vi "古田户外一体站流程质控自动启动.vi"(6 "CODMn量程切换":enum32{"H", "L", "AUTO"}(ring)=enum."AUTO", 8 "总磷量程切换":enum32{"H", "L", "AUTO"}(ring)=enum."AUTO", 9 "总氮量程切换":enum32{"H", "L", "AUTO"}(ring)=enum."AUTO", 10 "氨氮量程切换":enum32{"H", "L", "AUTO"}(ring)=enum."AUTO", 11 "参数":T1={"是否启用仪器"=FALSE, "CODMn"={"启动测量模式"={"测量模式"=enum."水样测量"}, "确定按钮"=TRUE}, "启动模块"={"氨氮"=FALSE, "总磷"=FALSE, "总氮"=FALSE, "COD"=FALSE}, "常规启动"=FALSE, "直接启动"=FALSE}) -> ()   [LabVIEW 2016, in "质控单元.lvlib"]
uses:
  PLC/PLC.lvlib
panel:
  out "枚举 2":enum16{"初始化", "采配水启动", "等待", "配水", "排水", "结束"}(ring)
  out "枚举":enum16{"初始化", "采配水启动", "等待", "配水", "排水", "结束"}(ring)
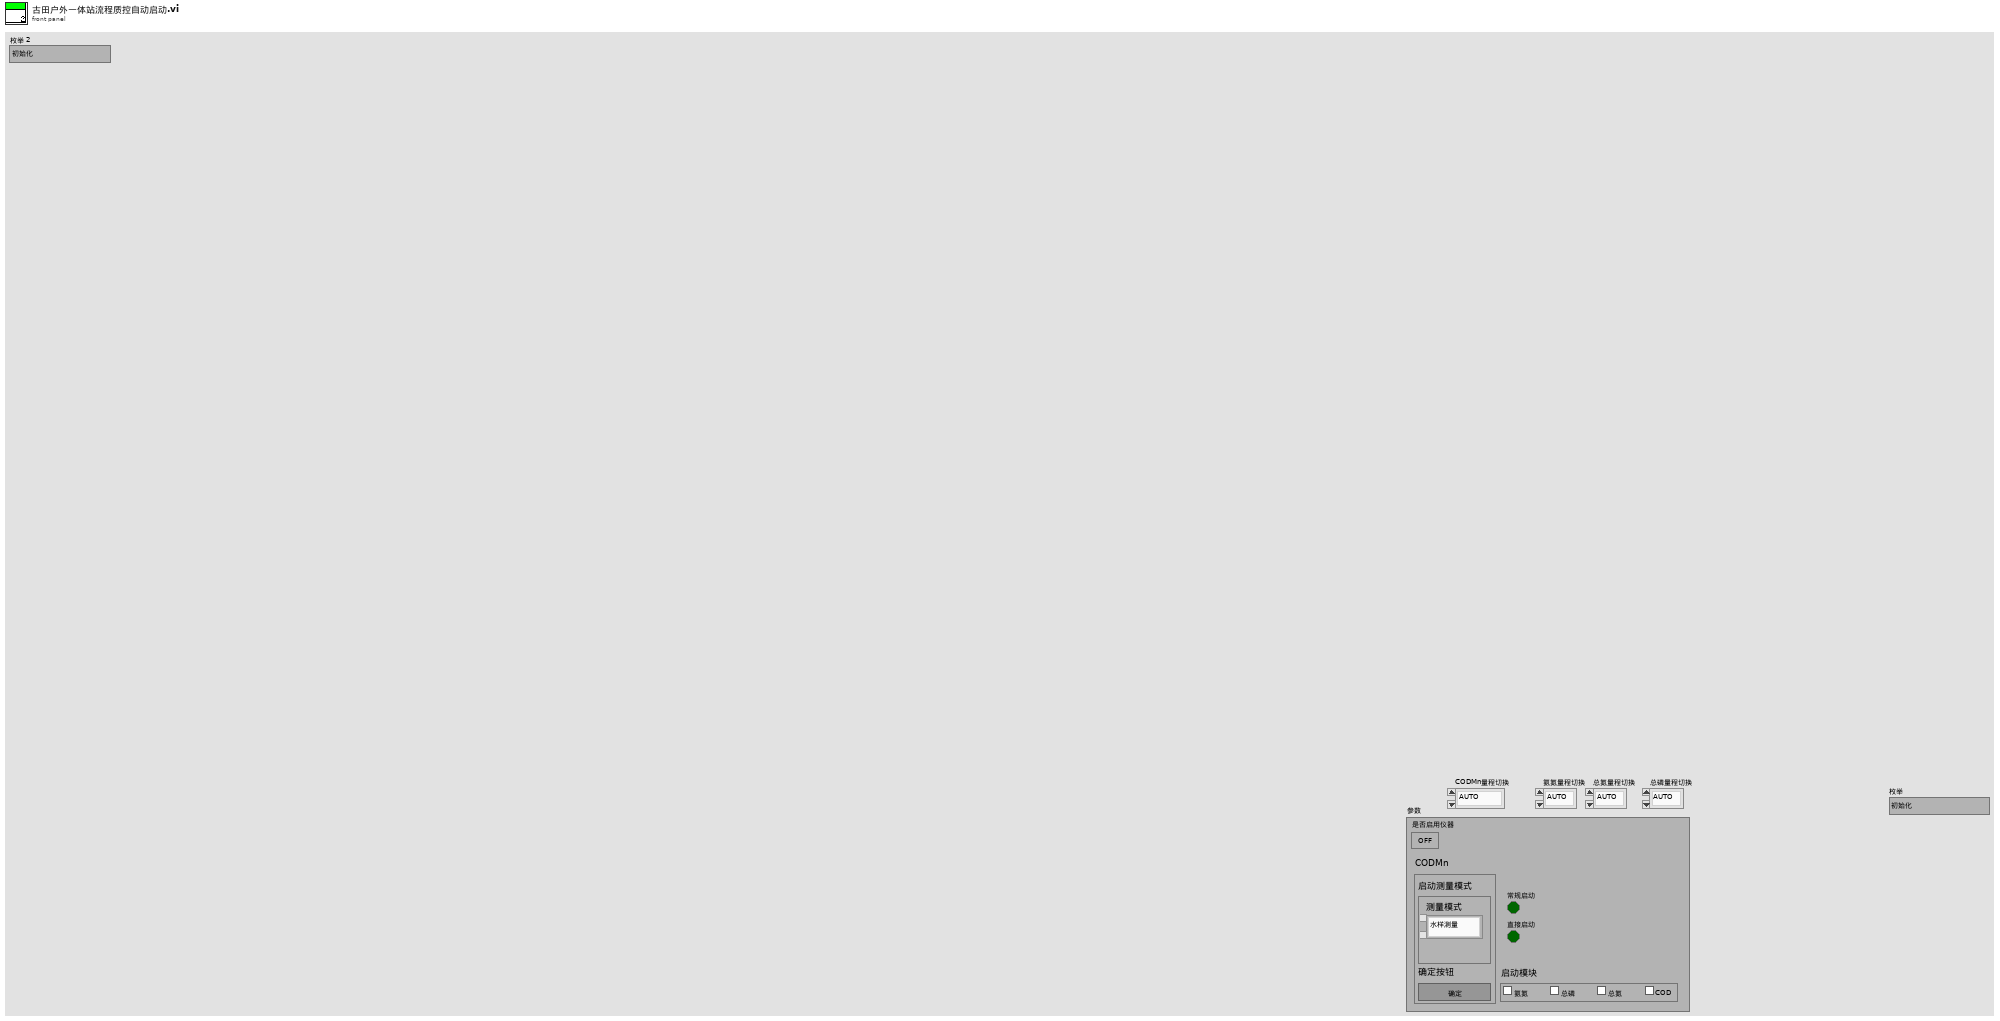
[diagram p1: front panel]
types:
  T1 = cluster{"是否启用仪器":bool, "CODMn":cluster{"启动测量模式":cluster{"测量模式":enum16{"水样测量", "标样核查", "加标回收", "平行样", "校零", "校标"}}, "确定按钮":bool}, "启动模块":cluster{"氨氮":bool, "总磷":bool, "总氮":bool, "COD":bool}, "常规启动":bool, "直接启动":bool}
  T2 = cluster{"命令":string, cluster{"starting address":u16, "holding register value":u16}}
  T3 = cluster{"R0":i16, "R1":i16, "R2":i16, "R3":i16, "R4":i16, "R5":i16, "R6":i16, "R7":i16, "R8":i16, "R9":i16, "R10":i16, "R11":i16, "R12":i16, "R13":i16, "R14":i16, "R15":i16, "R16":i16, "R17":i16, "R18":i16, "R19":i16, "R20":i16, "R21":i16, "R22":i16, "R23":i16, "R24":i16, "R25":i16}
  T4 = enum32{"Bad", "Idle", "Run top level", "Running"}
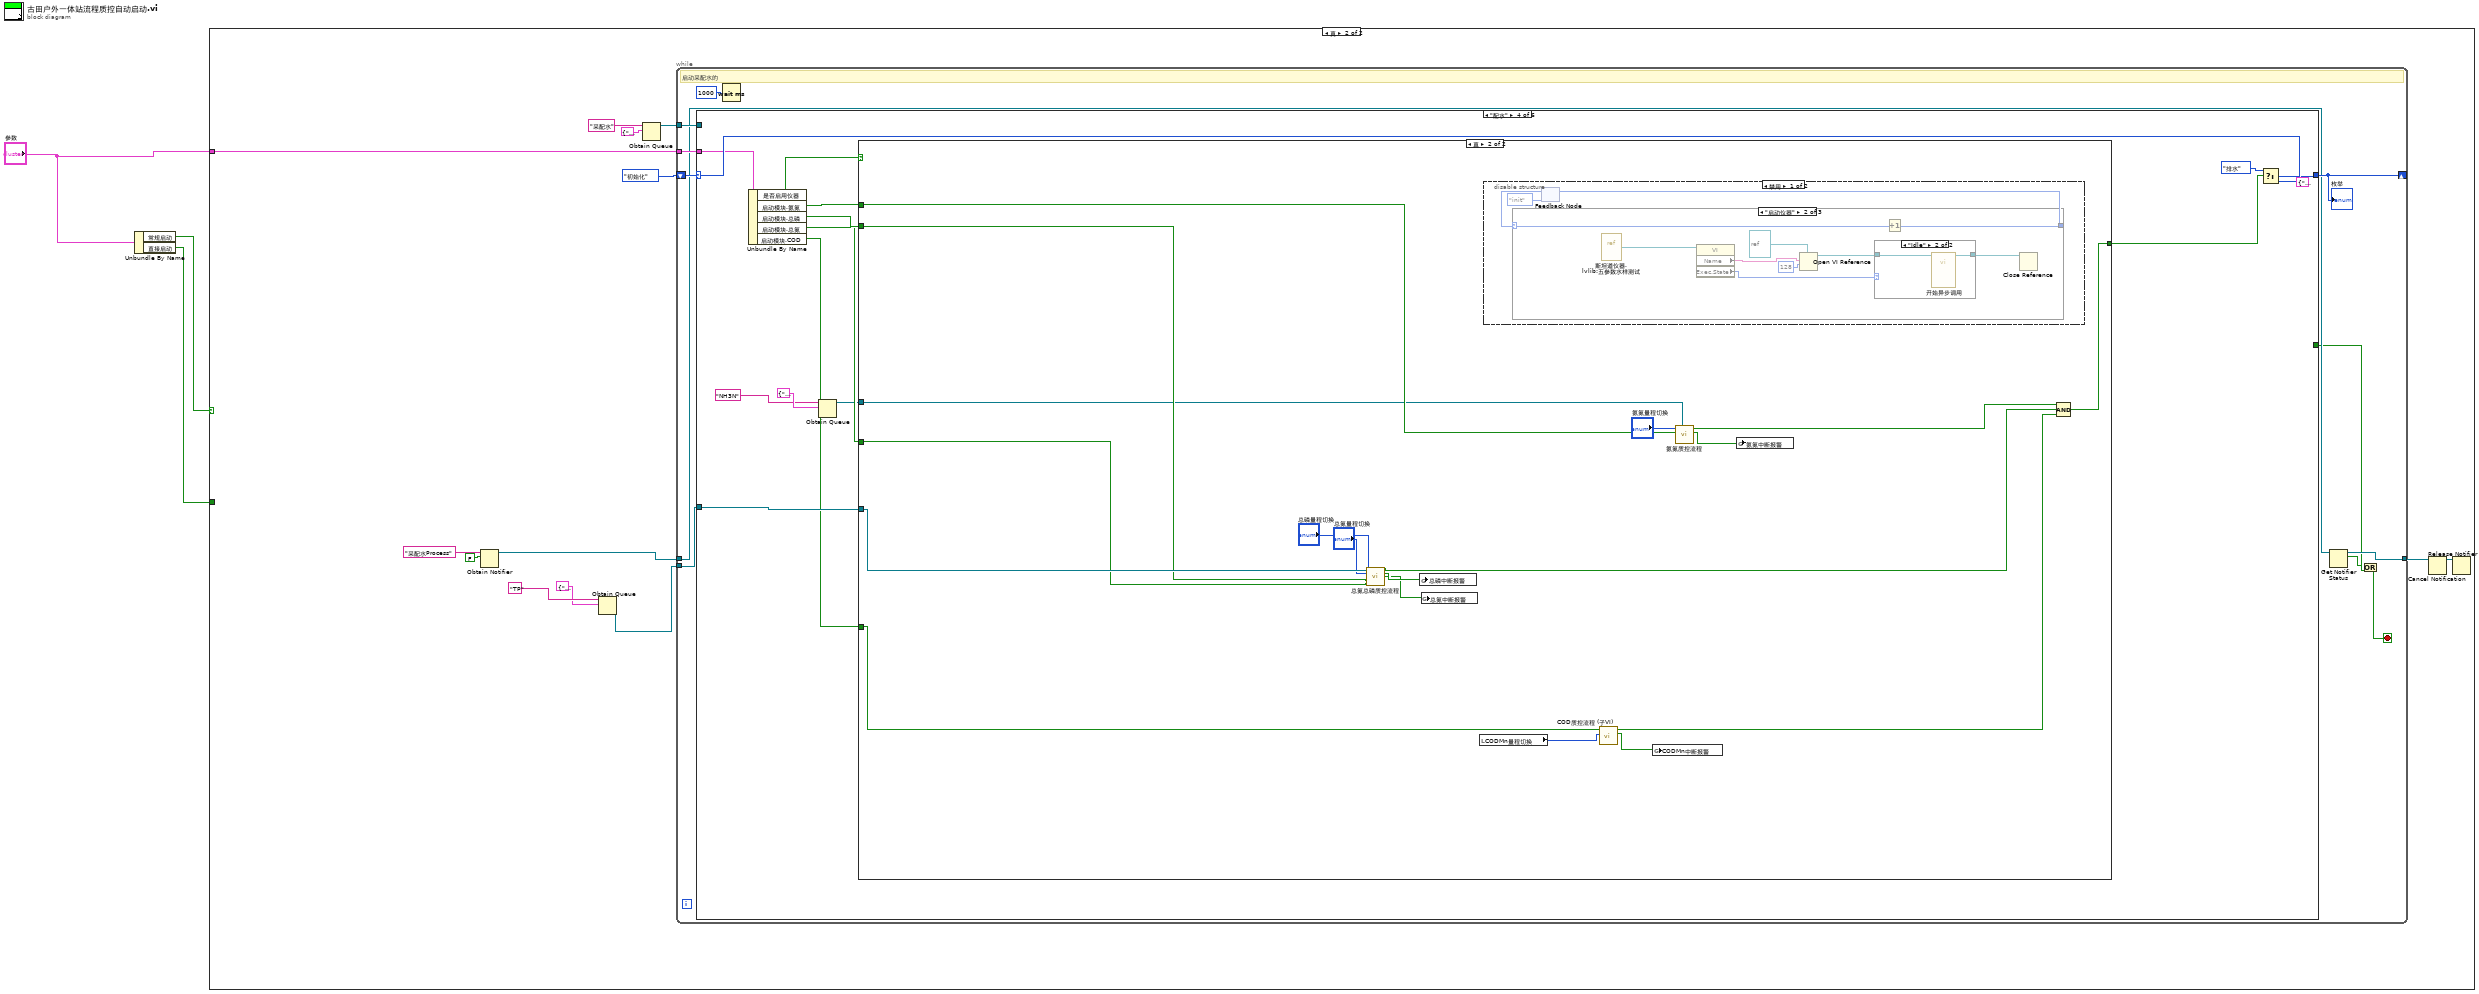
[diagram p0: block diagram]
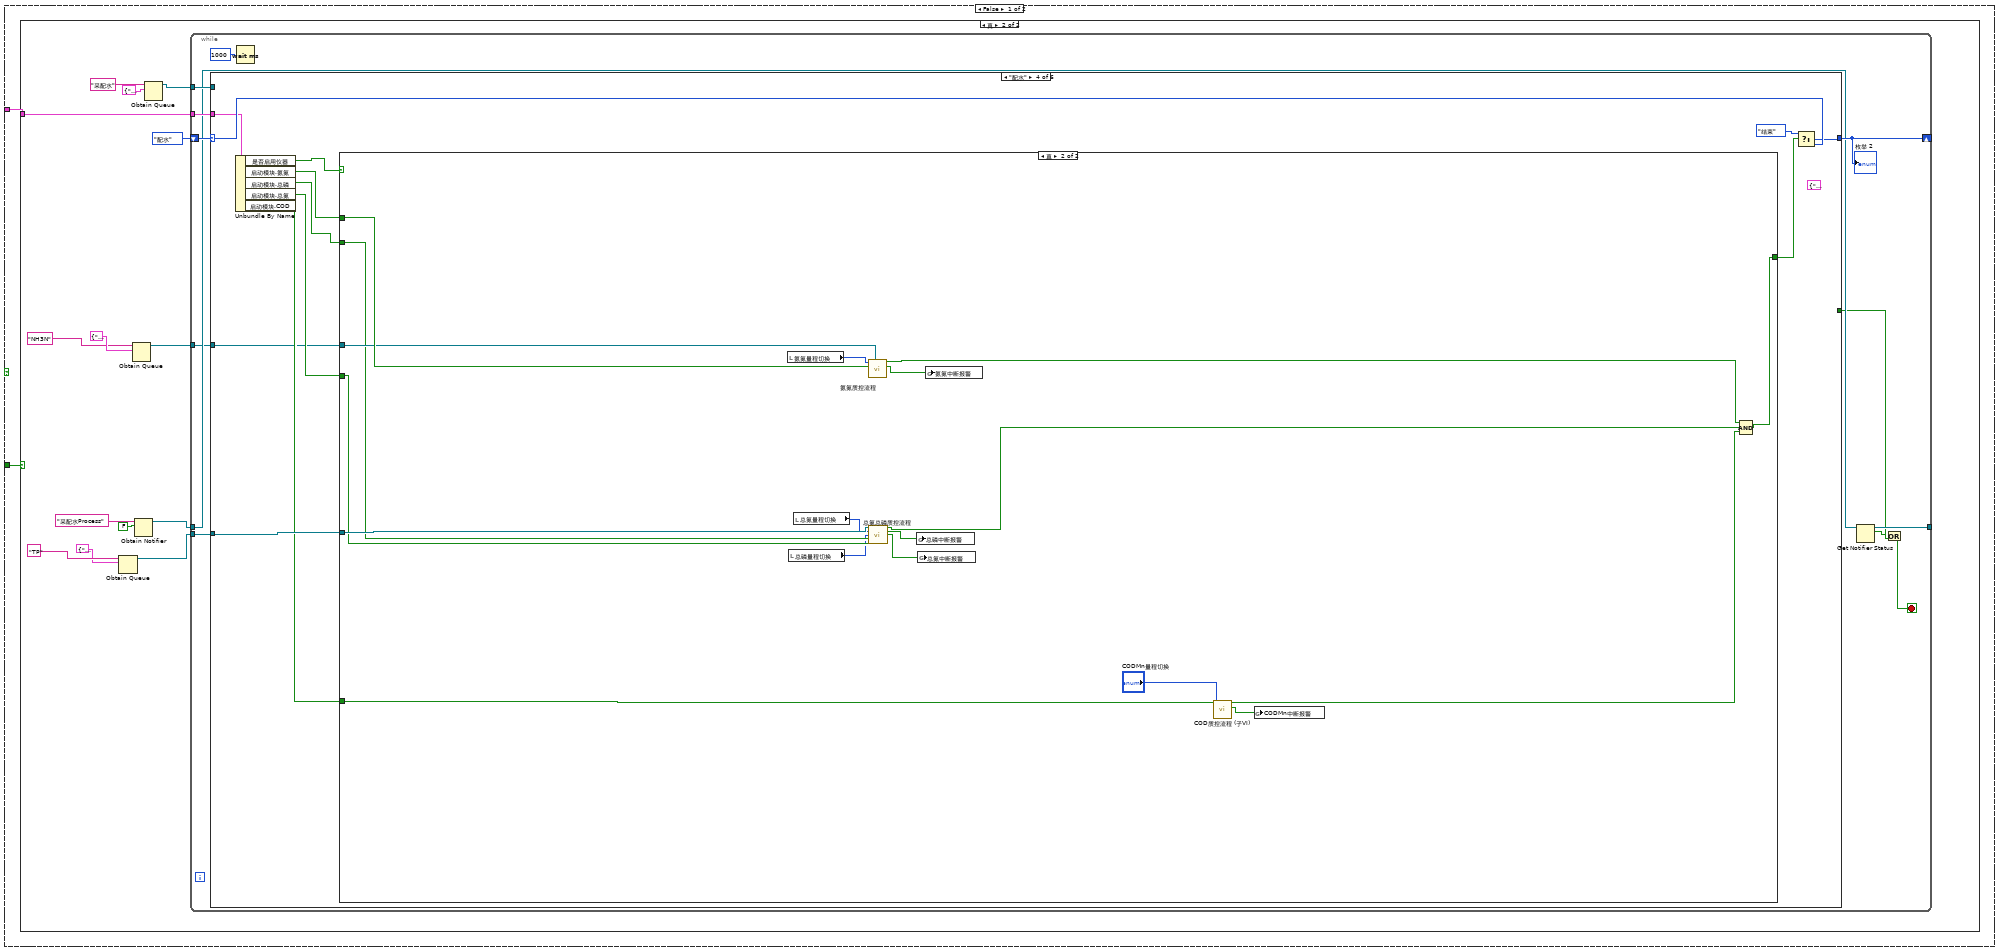
[diagram p2: hidden frame]
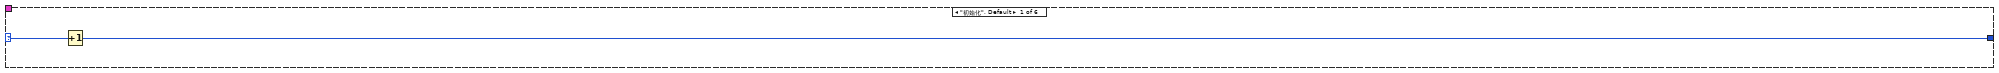
[diagram p4: hidden frame]
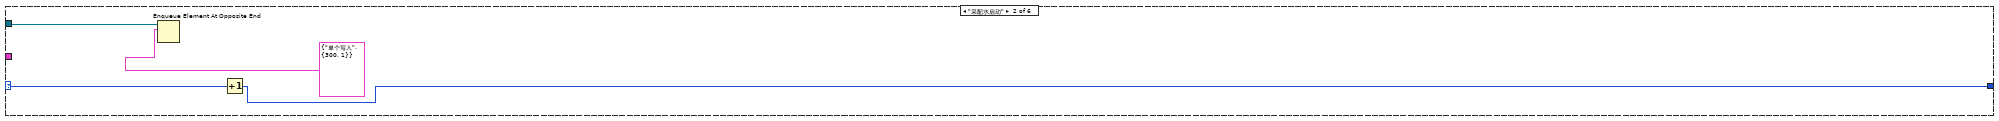
[diagram p5: hidden frame]
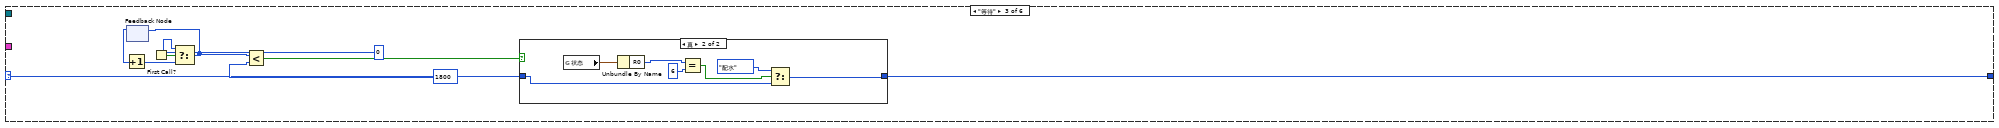
[diagram p6: hidden frame]
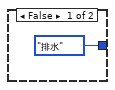
[diagram p7: hidden frame]
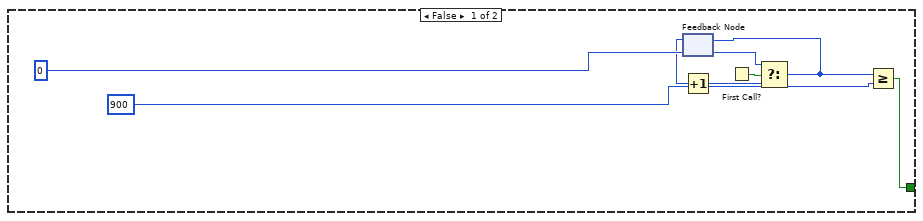
[diagram p8: hidden frame]
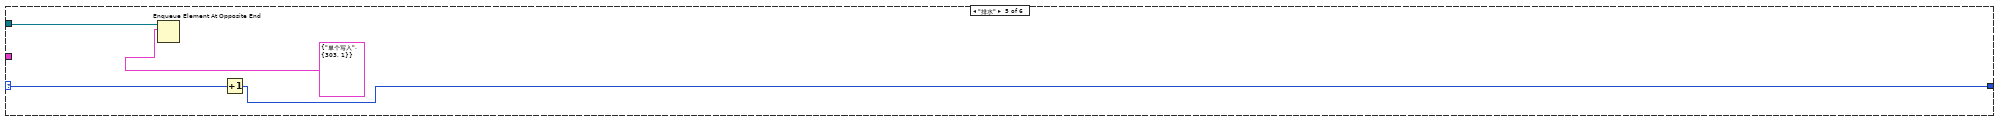
[diagram p9: hidden frame]
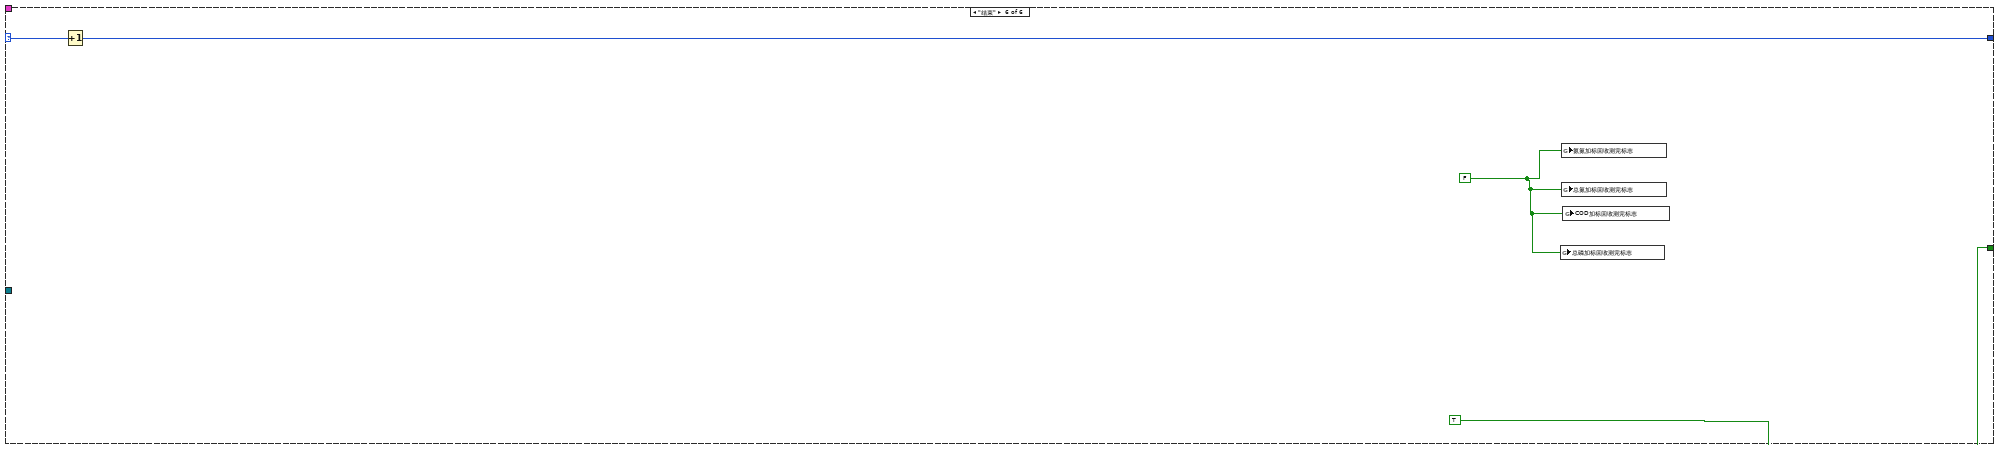
[diagram p10: hidden frame]
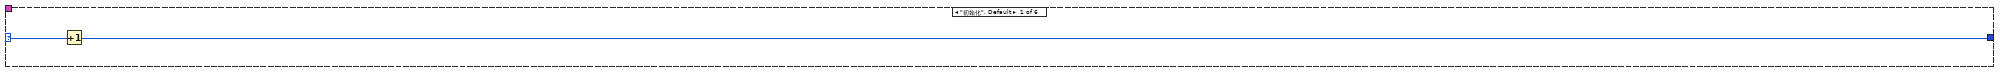
[diagram p11: hidden frame]
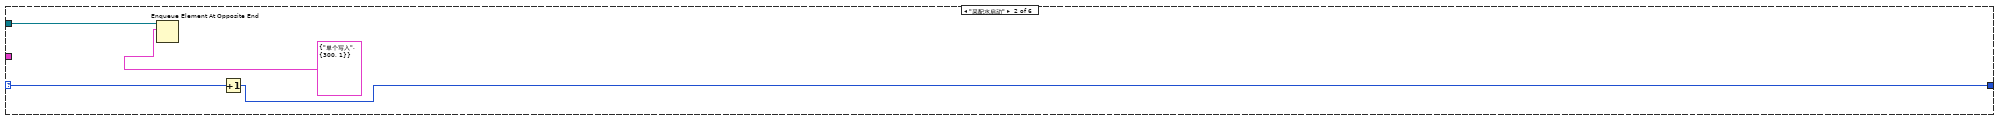
[diagram p12: hidden frame]
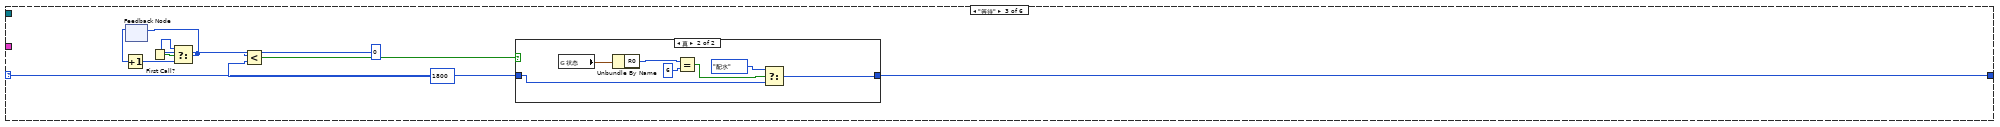
[diagram p13: hidden frame]
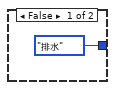
[diagram p14: hidden frame]
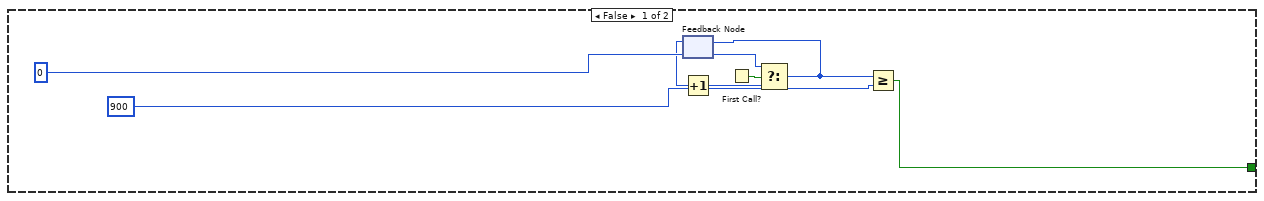
[diagram p15: hidden frame]
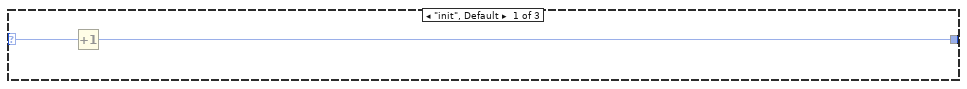
[diagram p16: hidden frame]
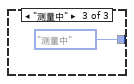
[diagram p18: hidden frame]
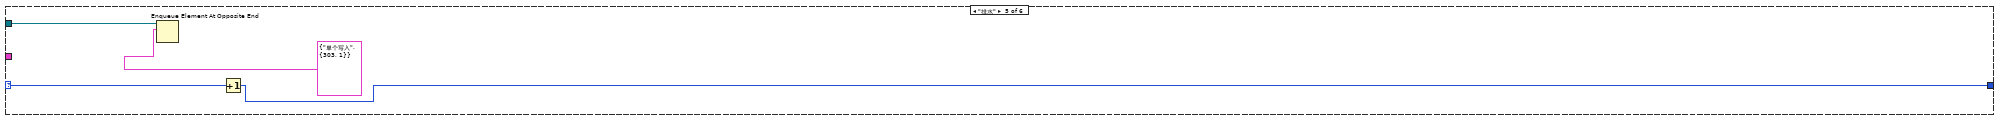
[diagram p20: hidden frame]
diagram:
  n1 = Unbundle By Name("参数") -> ("常规启动"=w2:bool, "直接启动"=w1:bool)
  n2 = case shown="真" w2 {
    tunnel: "参数" -> [w4 w100]
    tunnel: w1 -> [w5 _]
    frame False {
      n3 = case shown="真" w5 {
        tunnel: w4 -> [_ w18]
        frame False {
        }
        frame True {
          n4 = Obtain Queue(name (unnamed)="TP" ("名称（未命名）"), element data type=cluster{"命令":string, "data":variant} {"命令"="", "data"=variant}) -> (queue out=w9:refnum<queue>)  [unwired: 3 in, 2 out]
          n5 = Obtain Queue(name (unnamed)="NH3N" ("名称（未命名）"), element data type=cluster{"命令":string, "data":variant} {"命令"="", "data"=variant}) -> (queue out=w6:refnum<queue>)  [unwired: 3 in, 2 out]
          n6 = Obtain Notifier(name (unnamed)="采配水Process" ("名称（未命名）"), notification data type=FALSE) -> (notifier out=w12:refnum<notifier>)  [unwired: 2 in, 2 out]
          n7 = Obtain Queue(name (unnamed)="采配水" ("名称（未命名）"), element data type=cluster{"命令":string, "数据":variant} {"命令"="", "数据"=variant}) -> (queue out=w15:refnum<queue>)  [unwired: 3 in, 2 out]
          n8 = while {
            tunnel: w15 -> [w31]
            shift-right: [w29] -> _
            shift-left: enum16{"初始化", "采配水启动", "等待", "配水", "排水", "结束"}."配水" ("枚举") -> [w30]
            tunnel: w9 -> [w27]
            tunnel: w18 -> [w26]
            tunnel: w12 -> [w25]
            tunnel: [w24] -> _
            tunnel: w6 -> [w20]
            stop <- w23 stop-if-true
            n9 = case shown="\"配水\"" w30 {
              selector: w30 -> [w33 w35 w44 w65 w93 w99]
              tunnel: w31 -> [_ w36 _ _ w94 _]
              tunnel: [w32 w34 w43 w64 w92 w98] -> w29
              tunnel: [_ _ _ _ _ TRUE] -> w22
              tunnel: w27 -> [_ _ _ w63 _ _]
              tunnel: w26 -> [_ _ _ w60 _ _]
              tunnel: w20 -> [_ _ _ w55 _ _]
              frame "初始化", Default {
                n10 = Increment(x=w33) -> (x+1=w32:enum16{"初始化", "采配水启动", "等待", "配水", "排水", "结束"})
              }
              frame "采配水启动" {
                n11 = Enqueue Element At Opposite End(queue=w36, element=T2 {"命令"="单个写入", {"starting address"=300, "holding register value"=1}} ("元素")) -> ()  [unwired: 2 in, 3 out]
                n12 = Increment(x=w35) -> (x+1=w34:enum16{"初始化", "采配水启动", "等待", "配水", "排水", "结束"})
              }
              frame "等待" {
                n13 = feedback #1() -> (w40:i32)  [unwired: 1 in]
                n14 = Increment(x=w40) -> (x+1=w39:i32)
                n15 = First Call?() -> (First Call?: T/F=w41:bool)
                n16 = Select(t=0, s=w41, f=w39) -> (s? t:f=w38:i32)
                n17 = feedback-in #1(w38) -> ()
                n18 = Less?(x=w38, y=1800) -> (x < y?=w45:bool)
                n19 = case shown="真" w45 {
                  tunnel: w44 -> [_ w49]
                  tunnel: [enum16{"初始化", "采配水启动", "等待", "配水", "排水", "结束"}."排水" ("枚举") w48] -> w43
                  frame False {
                  }
                  frame True {
                    n20 = global read "采配水全局变量.vi" "状态"() -> (w54:T3)
                    n21 = Unbundle By Name(w54) -> ("R0"=w53:i16)
                    n22 = Equal?(x=w53, y=i16 6) -> (x = y?=w51:bool)
                    n23 = Select(t=enum16{"初始化", "采配水启动", "等待", "配水", "排水", "结束"}."配水" ("枚举"), s=w51, f=w49) -> (s? t:f=w48:enum16{"初始化", "采配水启动", "等待", "配水", "排水", "结束"})
                  }
                }
              }
              frame "配水" {
                (unwired) cluster{"命令":string, "data":variant} {"命令"="启动", "data"=variant(cluster{"站号":u16, "控制命令输出":u16[]} {"站号"=1, "控制命令输出"=[256, 0]})} ("元素")
                n24 = Unbundle By Name(w60) -> ("是否启用仪器"=w62:bool, "启动模块.氨氮"=w58:bool, "启动模块.总磷"=w59:bool, "启动模块.总氮"=w56:bool, "启动模块.COD"=w57:bool)
                n25 = case shown="真" w62 {
                  tunnel: w63 -> [_ w85]
                  tunnel: [w67 w91] -> w61
                  tunnel: w59 -> [_ w84]
                  tunnel: w58 -> [_ w90]
                  tunnel: w57 -> [_ w89]
                  tunnel: w56 -> [_ w83]
                  tunnel: w55 -> [_ w87]
                  frame False {
                    n26 = feedback #2() -> (w71:i32)  [unwired: 1 in]
                    n27 = Increment(x=w71) -> (x+1=w70:i32)
                    n28 = First Call?() -> (First Call?: T/F=w72:bool)
                    n29 = Select(t=0, s=w72, f=w70) -> (s? t:f=w68:i32)
                    n30 = feedback-in #2(w68) -> ()
                    n31 = Greater Or Equal?(x=w68, y=900) -> (x >= y?=w67:bool)
                  }
                  frame True {
                    n32 = local read "氨氮量程切换"() -> (w79:enum32{"H", "L", "AUTO"})
                    n33 = local read "总磷量程切换"() -> (w81:enum32{"H", "L", "AUTO"})
                    n34 = local read "总氮量程切换"() -> (w80:enum32{"H", "L", "AUTO"})
                    n35 = call "氨氮质控流程.vi"("队列输入NH3"=w87, "氨氮"=w90, "氨氮量程切换"=w79) -> ("氨氮中断报警"=w77:bool, "布尔"=w88:bool)  [unwired: 7 in]
                    n36 = call "总氮总磷质控流程.vi"("队列输入TP"=w85, "总氮量程切换"=w80, "总磷量程切换"=w81, "总磷"=w84, "总氮"=w83) -> ("布尔"=w82:bool, "总磷中断报警"=w76:bool, "总氮中断报警"=w75:bool)  [unwired: 8 in]
                    n37 = global write "质控中断报警全局.vi" "总磷中断报警"(w76) -> ()
                    n38 = global write "质控中断报警全局.vi" "总氮中断报警"(w75) -> ()
                    n39 = global write "质控中断报警全局.vi" "氨氮中断报警"(w77) -> ()
                    n40 = call "COD质控流程 (子VI).vi"("CODMn量程切换"="CODMn量程切换", "COD"=w89) -> ("CODMn中断报警"=w74:bool, "布尔"=w86:bool)  [unwired: 8 in]
                    n41 = global write "质控中断报警全局.vi" "CODMn中断报警"(w74) -> ()
                    n42 = Compound Arithmetic op=AND ("复合运算")(w88, w82, w86) -> (w91:bool)
                  }
                }
                n43 = Select(t=enum16{"初始化", "采配水启动", "等待", "配水", "排水", "结束"}."结束" ("枚举"), s=w61, f=w65) -> (s? t:f=w64:enum16{"初始化", "采配水启动", "等待", "配水", "排水", "结束"})
              }
              frame "排水" {
                n44 = Enqueue Element At Opposite End(queue=w94, element=T2 {"命令"="单个写入", {"starting address"=303, "holding register value"=1}} ("元素")) -> ()  [unwired: 2 in, 3 out]
                n45 = Increment(x=w93) -> (x+1=w92:enum16{"初始化", "采配水启动", "等待", "配水", "排水", "结束"})
              }
              frame "结束" {
                w96 = FALSE ("氨氮加标回收测完标志")
                n46 = Increment(x=w99) -> (x+1=w98:enum16{"初始化", "采配水启动", "等待", "配水", "排水", "结束"})
                n47 = global write "质控测完标志全局 1.vi" "总磷加标回收测完标志"(w96) -> ()
                n48 = global write "质控测完标志全局 1.vi" "氨氮加标回收测完标志"(w96) -> ()
                n49 = global write "质控测完标志全局 1.vi" "总氮加标回收测完标志"(w96) -> ()
                n50 = global write "质控测完标志全局 1.vi" "COD加标回收测完标志"(w96) -> ()
              }
            }
            "枚举 2" <- w29
            n51 = Wait (ms)(milliseconds to wait=u32 1000 ("等待时间（毫秒）")) -> ()  [unwired: 1 out]
            n52 = Get Notifier Status(notifier=w25) -> (notifier out=w24:refnum<notifier>, current notification=w21:bool)  [unwired: 1 in, 3 out]
            n53 = Or(x=w21, y=w22) -> (x .or. y?=w23:bool)
          }
        }
      }
    }
    frame True {
      n54 = Obtain Notifier(name (unnamed)="采配水Process" ("名称（未命名）"), notification data type=FALSE) -> (notifier out=w103:refnum<notifier>)  [unwired: 2 in, 2 out]
      n55 = Obtain Queue(name (unnamed)="TP" ("名称（未命名）"), element data type=cluster{"命令":string, "data":variant} {"命令"="", "data"=variant}) -> (queue out=w106:refnum<queue>)  [unwired: 3 in, 2 out]
      n56 = Obtain Queue(name (unnamed)="采配水" ("名称（未命名）"), element data type=cluster{"命令":string, "数据":variant} {"命令"="", "数据"=variant}) -> (queue out=w110:refnum<queue>)  [unwired: 3 in, 2 out]
      n57 = while {
        tunnel: w110 -> [w123]
        shift-right: [w121] -> _
        shift-left: enum16{"初始化", "采配水启动", "等待", "配水", "排水", "结束"}."初始化" ("枚举") -> [w122]
        tunnel: w106 -> [w119]
        tunnel: w100 -> [w118]
        tunnel: w103 -> [w117]
        tunnel: [w116] -> w102
        stop <- w115 stop-if-true
        # "启动采配水的"
        n58 = case shown="\"配水\"" w122 {
          selector: w122 -> [w125 w127 w136 w159 w205 w210]
          tunnel: w123 -> [_ w128 _ _ w206 _]
          tunnel: [w124 w126 w135 w158 w204 w209] -> w121
          tunnel: [_ _ _ _ _ TRUE] -> w114
          tunnel: w119 -> [_ _ _ w157 _ _]
          tunnel: w118 -> [_ _ _ w154 _ _]
          frame "初始化", Default {
            n59 = Increment(x=w125) -> (x+1=w124:enum16{"初始化", "采配水启动", "等待", "配水", "排水", "结束"})
          }
          frame "采配水启动" {
            n60 = Enqueue Element At Opposite End(queue=w128, element=T2 {"命令"="单个写入", {"starting address"=300, "holding register value"=1}} ("元素")) -> ()  [unwired: 2 in, 3 out]
            n61 = Increment(x=w127) -> (x+1=w126:enum16{"初始化", "采配水启动", "等待", "配水", "排水", "结束"})
          }
          frame "等待" {
            n62 = feedback #3() -> (w132:i32)  [unwired: 1 in]
            n63 = Increment(x=w132) -> (x+1=w131:i32)
            n64 = First Call?() -> (First Call?: T/F=w133:bool)
            n65 = Select(t=0, s=w133, f=w131) -> (s? t:f=w130:i32)
            n66 = feedback-in #3(w130) -> ()
            n67 = Less?(x=w130, y=1800) -> (x < y?=w137:bool)
            n68 = case shown="真" w137 {
              tunnel: w136 -> [_ w141]
              tunnel: [enum16{"初始化", "采配水启动", "等待", "配水", "排水", "结束"}."排水" ("枚举") w140] -> w135
              frame False {
              }
              frame True {
                n69 = global read "采配水全局变量.vi" "状态"() -> (w146:T3)
                n70 = Unbundle By Name(w146) -> ("R0"=w145:i16)
                n71 = Equal?(x=w145, y=i16 6) -> (x = y?=w143:bool)
                n72 = Select(t=enum16{"初始化", "采配水启动", "等待", "配水", "排水", "结束"}."配水" ("枚举"), s=w143, f=w141) -> (s? t:f=w140:enum16{"初始化", "采配水启动", "等待", "配水", "排水", "结束"})
              }
            }
          }
          frame "配水" {
            (unwired) cluster{"命令":string, "data":variant} {"命令"="启动", "data"=variant(cluster{"站号":u16, "控制命令输出":u16[]} {"站号"=1, "控制命令输出"=[256, 0]})} ("元素")
            n73 = Unbundle By Name(w154) -> ("是否启用仪器"=w156:bool, "启动模块.氨氮"=w152:bool, "启动模块.总磷"=w153:bool, "启动模块.总氮"=w150:bool, "启动模块.COD"=w151:bool)
            n74 = Obtain Queue(name (unnamed)="NH3N" ("名称（未命名）"), element data type=cluster{"命令":string, "data":variant} {"命令"="", "data"=variant}) -> (queue out=w147:refnum<queue>)  [unwired: 3 in, 2 out]
            n75 = case shown="真" w156 {
              tunnel: w157 -> [_ w180]
              tunnel: [w161 w184] -> w155
              tunnel: w153 -> [_ w179]
              tunnel: w152 -> [_ w183]
              tunnel: w151 -> [_ w182]
              tunnel: w150 -> [_ w178]
              tunnel: w147 -> [_ w174]
              frame False {
                n76 = feedback #4() -> (w165:i32)  [unwired: 1 in]
                n77 = Increment(x=w165) -> (x+1=w164:i32)
                n78 = First Call?() -> (First Call?: T/F=w166:bool)
                n79 = Select(t=0, s=w166, f=w164) -> (s? t:f=w162:i32)
                n80 = feedback-in #4(w162) -> ()
                n81 = Greater Or Equal?(x=w162, y=900) -> (x >= y?=w161:bool)
              }
              frame True {
                n82 = call "总氮总磷质控流程.vi"("队列输入TP"=w180, "总氮量程切换"="总氮量程切换", "总磷量程切换"="总磷量程切换", "总磷"=w179, "总氮"=w178) -> ("布尔"=w177:bool, "总磷中断报警"=w170:bool, "总氮中断报警"=w169:bool)  [unwired: 8 in]
                n83 = global write "质控中断报警全局.vi" "总磷中断报警"(w170) -> ()
                n84 = global write "质控中断报警全局.vi" "总氮中断报警"(w169) -> ()
                n85 = local read "CODMn量程切换"() -> (w172:enum32{"H", "L", "AUTO"})
                n86 = disable-structure shown="禁用" {
                  frame Disabled {
                    n87 = feedback #5(enum16{"init", "启动仪器", "测量中"}."init") -> (w187:enum16{"init", "启动仪器", "测量中"})
                    n88 = case shown="\"启动仪器\"" w187 {
                      selector: w187 -> [w190 w199 _]
                      tunnel: [w189 w198 enum16{"init", "启动仪器", "测量中"}."测量中"] -> w188
                      frame "init", Default {
                        n89 = Increment(x=w190) -> (x+1=w189:enum16{"init", "启动仪器", "测量中"})
                      }
                      frame "启动仪器" {
                        n90 = vi-ref "斯坦道仪器.lvlib:五参数水样测试.vi"() -> (w191:refnum<vi>)
                        n91 = property class="VI"(reference=w191) -> ("Name"=w195:string, "Exec.State"=w193:T4)  [unwired: 1 in, 2 out]
                        n92 = Open VI Reference(type specifier VI Refnum (for type only)=refnum<vi> refnum ("类型说明符VI引用句柄（仅用于类型）"), vi path=w195, options=128 ("选项")) -> (vi reference=w194:refnum<vi>)  [unwired: 3 in, 1 out]
                        n93 = case shown="\"Idle\"" w193 {
                          tunnel: w194 -> [w200 w202]
                          tunnel: [w200 w201] -> w192
                          frame "Bad", Default {
                          }
                          frame "Idle" {
                            n94 = call-by-ref "开始异步调用"(reference=w202) -> (reference out=w201:refnum<vi>)  [unwired: 13 in, 1 out]
                          }
                        }
                        n95 = Increment(x=w199) -> (x+1=w198:enum16{"init", "启动仪器", "测量中"})
                        n96 = Close Reference(reference=w192) -> ()  [unwired: 1 in, 1 out]
                      }
                      frame "测量中" {
                      }
                    }
                    n97 = feedback-in #5(w188) -> ()
                  }
                  frame Enabled {
                  }
                }
                n98 = call "COD质控流程 (子VI).vi"("CODMn量程切换"=w172, "COD"=w182) -> ("CODMn中断报警"=w171:bool, "布尔"=w181:bool)  [unwired: 8 in]
                n99 = global write "质控中断报警全局.vi" "CODMn中断报警"(w171) -> ()
                n100 = call "氨氮质控流程.vi"("队列输入NH3"=w174, "氨氮"=w183, "氨氮量程切换"="氨氮量程切换") -> ("氨氮中断报警"=w168:bool, "布尔"=w185:bool)  [unwired: 7 in]
                n101 = global write "质控中断报警全局.vi" "氨氮中断报警"(w168) -> ()
                n102 = Compound Arithmetic op=AND ("复合运算")(w185, w177, w181) -> (w184:bool)
              }
            }
            n103 = Select(t=enum16{"初始化", "采配水启动", "等待", "配水", "排水", "结束"}."排水" ("枚举"), s=w155, f=w159) -> (s? t:f=w158:enum16{"初始化", "采配水启动", "等待", "配水", "排水", "结束"})
          }
          frame "排水" {
            n104 = Enqueue Element At Opposite End(queue=w206, element=T2 {"命令"="单个写入", {"starting address"=303, "holding register value"=1}} ("元素")) -> ()  [unwired: 2 in, 3 out]
            n105 = Increment(x=w205) -> (x+1=w204:enum16{"初始化", "采配水启动", "等待", "配水", "排水", "结束"})
          }
          frame "结束" {
            n106 = Increment(x=w210) -> (x+1=w209:enum16{"初始化", "采配水启动", "等待", "配水", "排水", "结束"})
          }
        }
        "枚举" <- w121
        n107 = Wait (ms)(milliseconds to wait=u32 1000 ("等待时间（毫秒）")) -> ()  [unwired: 1 out]
        n108 = Get Notifier Status(notifier=w117) -> (notifier out=w116:refnum<notifier>, current notification=w113:bool)  [unwired: 1 in, 3 out]
        n109 = Or(x=w113, y=w114) -> (x .or. y?=w115:bool)
      }
      n110 = Cancel Notification(0:w102) -> (8:w101:refnum<notifier>)  [unwired: 1 in, 2 out]
      n111 = Release Notifier(notifier=w101) -> ()  [unwired: 2 in, 3 out]
    }
  }
